vi "Engage Set Screw 2.vi"(0 "reference in":refnum<class "SmartMotor.lvclass">, 5 "error in (no error)":errorcluster) -> (14 "reference out":refnum<class "SmartMotor.lvclass">, 18 "Screw Engaged":bool, 19 "error out":errorcluster)   [LabVIEW 2017]
uses:
  SmartMotor.lvclass
panel:
  in  "Number of Tries":i32=2
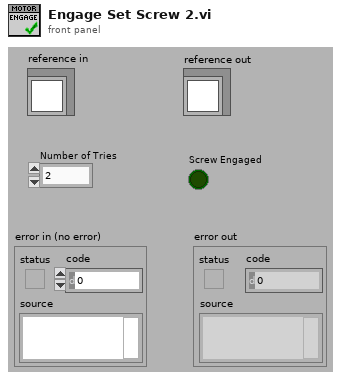
[diagram p1: front panel]
types:
  T1 = typedef "SmartMotor.lvclass/ObjectAttributes.ctl" = cluster{"SmartMotor Chain VISA Resource":refnum<visa-resource-name>, "SmartMotor Chain Address":i16, "Motor Absolute Position":i32, "Motor Relative Position":i32, "Motor Torque":i32, "Motor Voltage":i32, "Screwdriver Engaged":bool, "Screwdriver Torque Limit":i32, "Torque Monitor On/Off Status":bool, "Torque Monitor VI Reference":refnum<vi>, "Absolute Motor Torque (Filtered)":dbl, "SmartMotor Status":T2, "SmartMotor Error":T3}
  T2 = typedef "SmartMotor.lvclass/SmartMotor Status.ctl" = enum8{"Stopped", "Moving"}
  T3 = typedef "SmartMotor.lvclass/SmartMotor Error.ctl" = enum8{"None", "Read Error", "Low Voltage"}
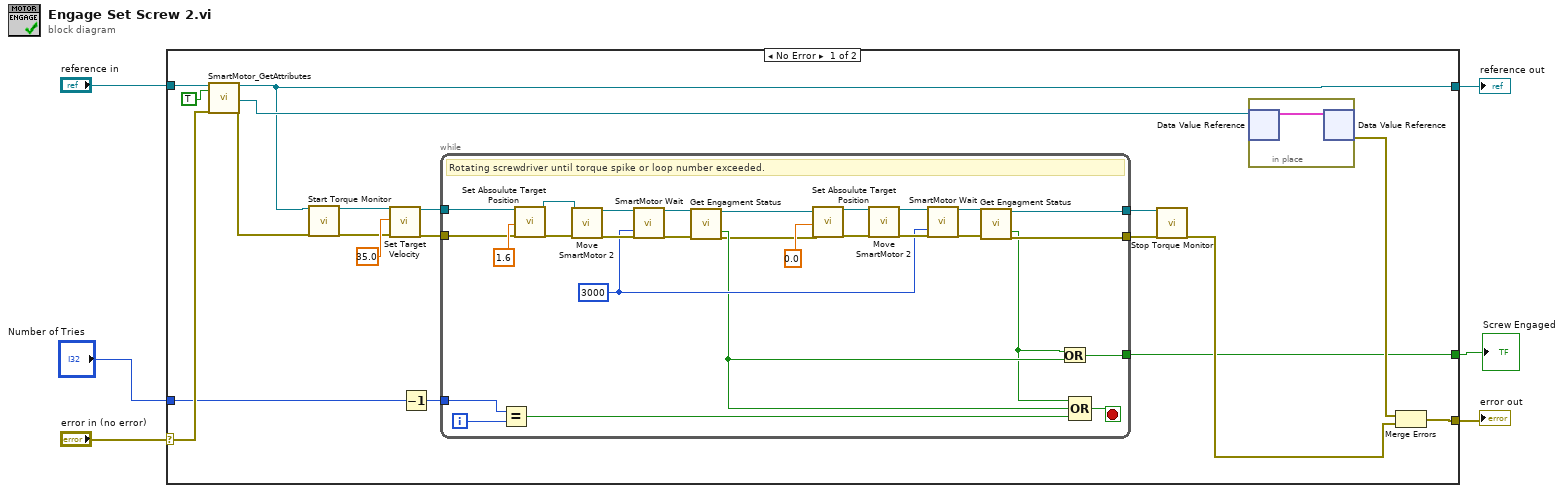
[diagram p0: block diagram]
diagram:
  n1 = case shown="No Error" "error in (no error)" {
    selector: "error in (no error)" -> [w24 w56]
    tunnel: [w22 w56] -> w5
    tunnel: [w17 w55] -> w3
    tunnel: "reference in" -> [w25 w55]
    tunnel: [w7 _] -> w2
    tunnel: "Number of Tries" -> [w18 _]
    frame No Error {
      n2 = call "SmartMotor_GetAttributes.vi"("reference in"=w25, "OnlyGetDvrReference(False)"=TRUE, "error in (no error)"=w24) -> ("reference out"=w17:refnum<class "SmartMotor.lvclass">, "DataRef"=w21:refnum<data-value>, "error out"=w12:errorcluster)  [unwired: 13 in, 1 out]
      n3 = call-dynamic "Start Torque Monitor.vi"("reference in"=w17, "error in (no error)"=w12) -> ("reference out"=w16:refnum<class "SmartMotor.lvclass">, "error out"=w13:errorcluster)  [unwired: 16 in]
      n4 = call-dynamic "Set Target Velocity.vi"("reference in"=w16, "Target Velocity (RPM)"=35.0, "error in (no error)"=w13) -> ("reference out"=w15:refnum<class "SmartMotor.lvclass">, "error out"=w14:errorcluster)  [unwired: 15 in]
      n5 = Decrement(x=w18) -> (x-1=w19:i32)
      n6 = while {
        tunnel: w15 -> [w48]
        tunnel: w14 -> [w46]
        tunnel: [w27] -> w10
        tunnel: [w42] -> w7
        tunnel: w19 -> [w41]
        tunnel: [w28] -> w11
        i -> [w45]
        stop <- w43 stop-if-true
        w36 = u32 3000 ("Number of Milliseconds to Wait")
        # "Rotating screwdriver until torque spike or loop number exceeded."
        n7 = Equal?(x=w41, y=w45) -> (x = y?=w44:bool)
        n8 = call-dynamic "Set Absoulute Target Position.vi"("reference in"=w48, "Absoulute Target Position (Revolutions)"=1.6, "error in (no error)"=w46) -> ("reference out"=w51:refnum<class "SmartMotor.lvclass">, "error out"=w50:errorcluster)  [unwired: 15 in]
        n9 = call-dynamic "Move SmartMotor 2.vi"("reference in"=w51, "error in (no error)"=w50) -> ("reference out"=w40:refnum<class "SmartMotor.lvclass">, "error out"=w39:errorcluster)  [unwired: 16 in]
        n10 = call-dynamic "SmartMotor Wait.vi"("reference in"=w40, "Number of Milliseconds to Wait"=w36, "error in (no error)"=w39) -> ("reference out"=w35:refnum<class "SmartMotor.lvclass">, "error out"=w32:errorcluster)  [unwired: 15 in]
        n11 = call-dynamic "Get Engagment Status.vi"("reference in"=w35, "error in (no error)"=w32) -> ("reference out"=w34:refnum<class "SmartMotor.lvclass">, "Screwdriver Engaged"=w33:bool, "error out"=w31:errorcluster)  [unwired: 15 in]
        n12 = call-dynamic "Set Absoulute Target Position.vi"("reference in"=w34, "Absoulute Target Position (Revolutions)"=0.0, "error in (no error)"=w31) -> ("reference out"=w53:refnum<class "SmartMotor.lvclass">, "error out"=w52:errorcluster)  [unwired: 15 in]
        n13 = call-dynamic "Move SmartMotor 2.vi"("reference in"=w53, "error in (no error)"=w52) -> ("reference out"=w38:refnum<class "SmartMotor.lvclass">, "error out"=w37:errorcluster)  [unwired: 16 in]
        n14 = call-dynamic "SmartMotor Wait.vi"("reference in"=w38, "Number of Milliseconds to Wait"=w36, "error in (no error)"=w37) -> ("reference out"=w30:refnum<class "SmartMotor.lvclass">, "error out"=w29:errorcluster)  [unwired: 15 in]
        n15 = call-dynamic "Get Engagment Status.vi"("reference in"=w30, "error in (no error)"=w29) -> ("reference out"=w28:refnum<class "SmartMotor.lvclass">, "Screwdriver Engaged"=w26:bool, "error out"=w27:errorcluster)  [unwired: 15 in]
        n16 = Or(x=w26, y=w33) -> (x .or. y?=w42:bool)
        n17 = Compound Arithmetic op=OR(w26, w33, w44) -> (w43:bool)
      }
      n18 = call-dynamic "Stop Torque Monitor.vi"("reference in"=w11, "error in (no error)"=w10) -> ("error out"=w9:errorcluster)  [unwired: 16 in, 1 out]
      n19 = in-place {
        n20 = in-place-dvr #1(w21) -> (w54:T1)  [unwired: 1 out]
        n21 = in-place-dvr #1(w54) -> (w23:errorcluster)  [unwired: 1 out]
      }
      n22 = Merge Errors(w23, w9) -> (w22:errorcluster)
    }
    frame Error {
    }
  }
  "error out" <- w5
  "reference out" <- w3
  "Screw Engaged" <- w2
